vi "main OP300.vi"() -> ()   [LabVIEW 2020]
uses:
  SubVI/OP300ZP_state.ctl
  <vilib>/Sylvain.lib/02 SLIM ZEN WS 500/SubVi/FGV.ctl
  <vilib>/Sylvain.lib/02 SLIM ZEN WS 500/SubVi/VG_progressBar.vi
  SubVI/CheminDeBase.vi
  VG/PN.vi
  VG/IS30%.vi
panel:
  out "IS30% ?":bool
  out "Cluster":T1
  out "VISA OUT":T2
  out "progression":u8(slide) scale=0.0..100.0
  out "PN":string
  out "errout 2":errorcluster={"status"=TRUE, "code"=0, "source"="PCAN_CHANNEL ILLEGAL"} caption="errout"
  out "errout":errorcluster caption="sortie d'erreur"
  out "STOP":bool
  out "TOP":string
  out "DRAW":picture
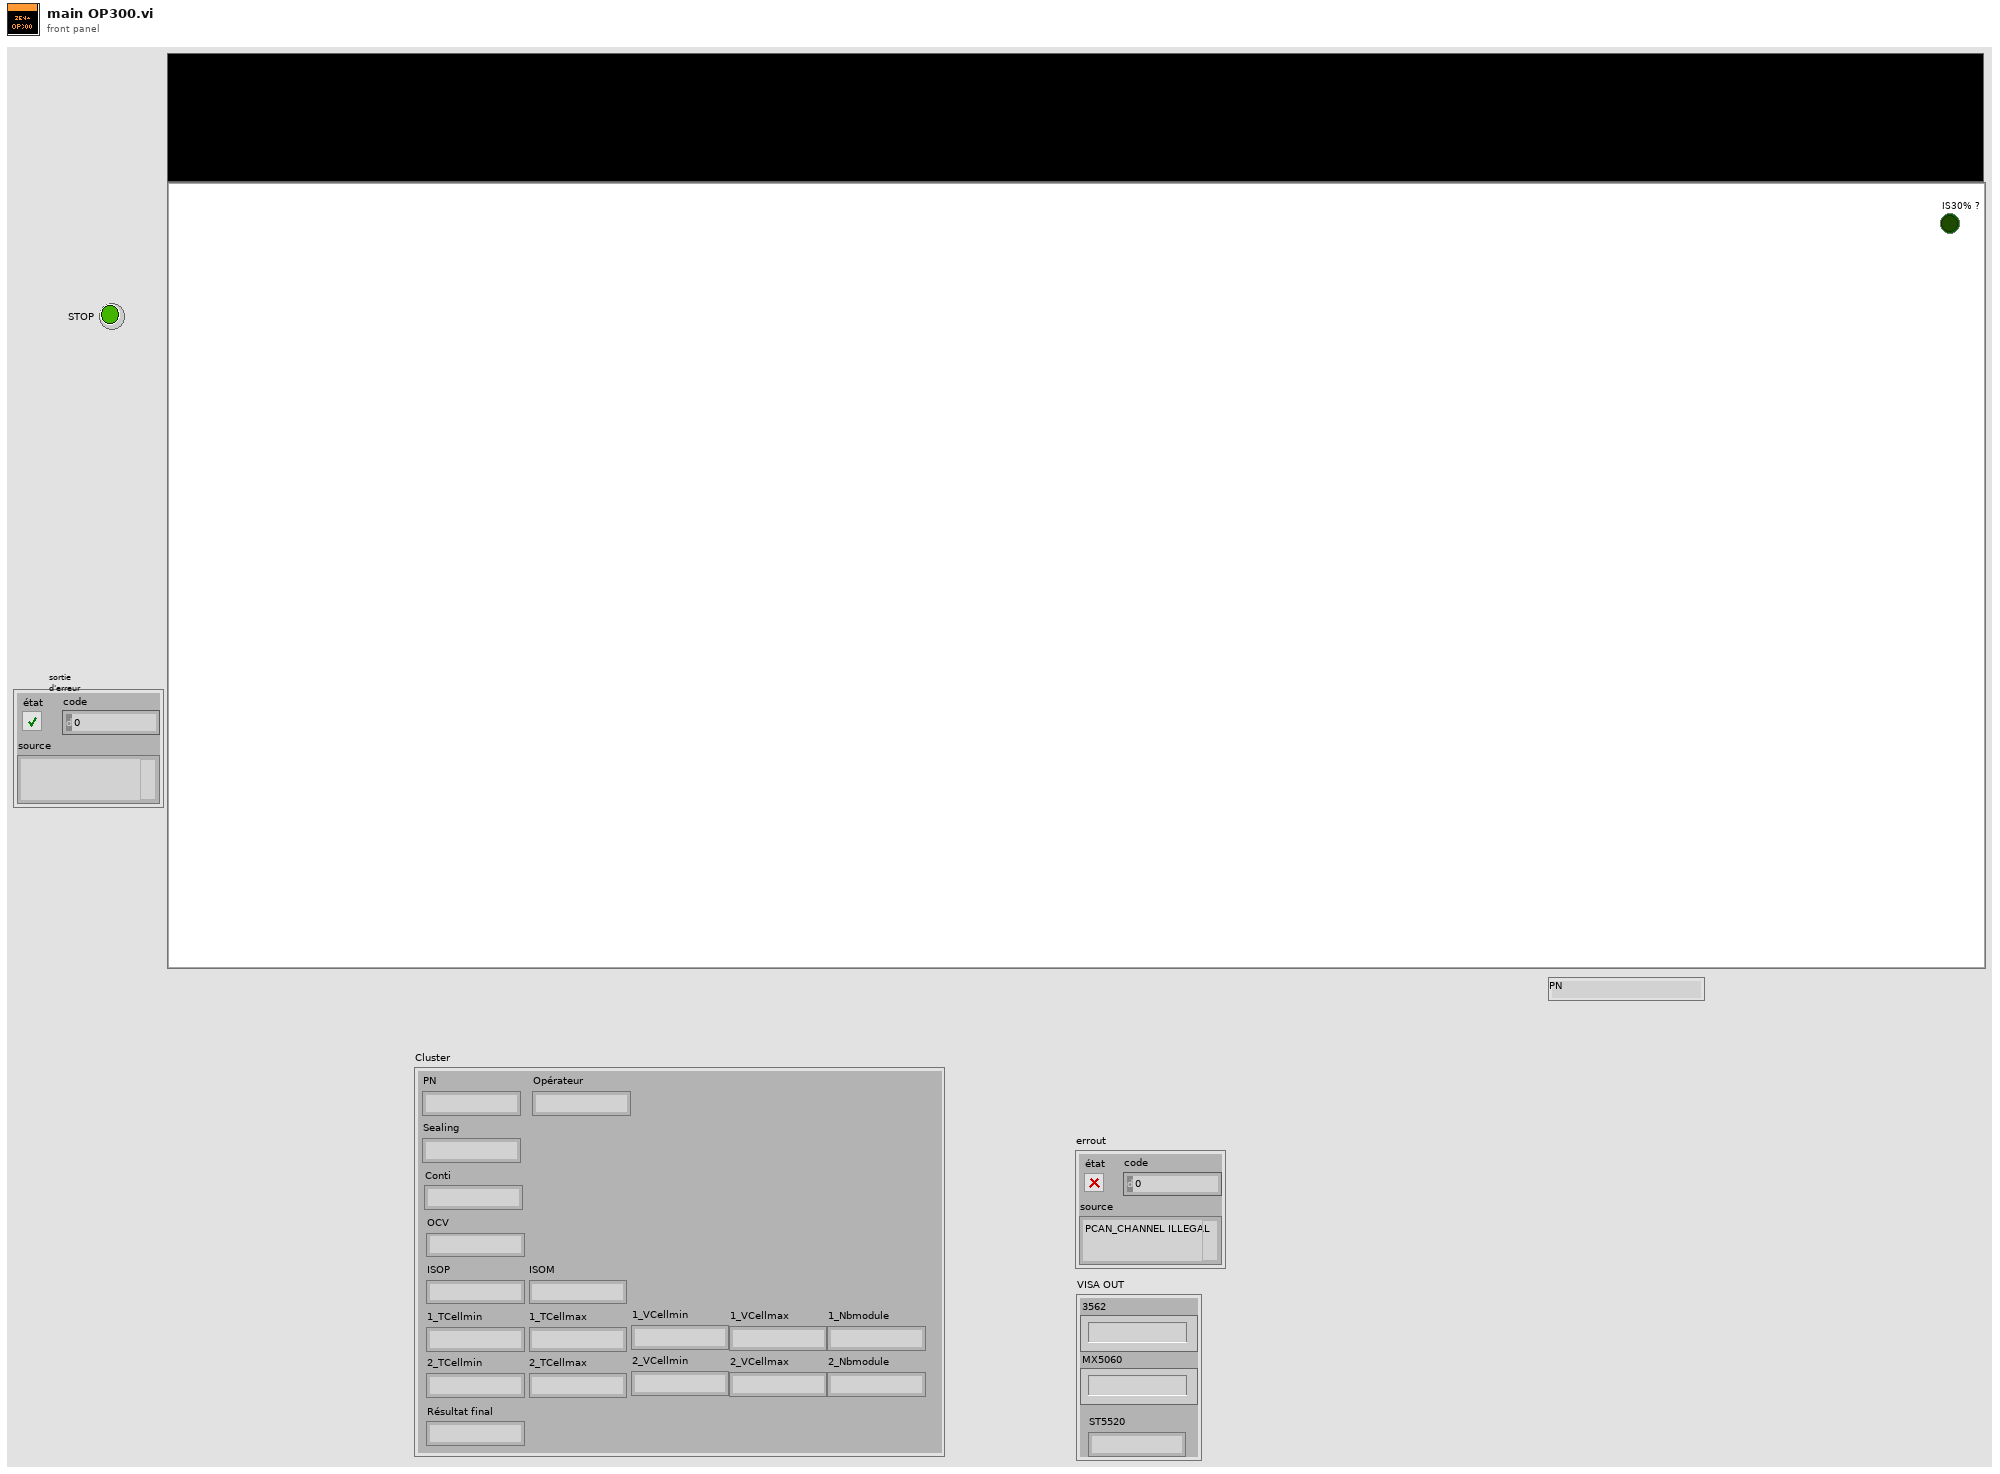
[diagram p1: front panel]
types:
  T1 = cluster{"PN":string, "Opérateur":string, "Sealing":string, "Conti":string, "OCV":string, "ISOP":string, "ISOM":string, "1_TCellmin":string, "1_TCellmax":string, "1_VCellmin":string, "1_VCellmax":string, "1_Nbmodule":string, "2_TCellmin":string, "2_TCellmax":string, "2_VCellmin":string, "2_VCellmax":string, "2_Nbmodule":string, "Résultat final":string}
  T2 = cluster{"3562":string, "MX5060":string, "ST5520":string}
  T3 = cluster{"PN":string, "Sealing":string, "Opérateur":string, "Conti":string, "OCV":string, "ISOP":string, "ISOM":string, "1_TCellmin":string, "1_TCellmax":string, "1_VCellmin":string, "1_VCellmax":string, "1_Nbmodule":string, "2_TCellmin":string, "2_TCellmax":string, "2_VCellmin":string, "2_VCellmax":string, "2_Nbmodule":string, "Résultat final":string}
  T4 = typedef "OP300ZP_state.ctl" = enum16{"Null", "Demarrage", "Init", "Scan", "Montage", "Conti", "OCV", "Iso", "Vpack", "DataDyn", "Dessouter", "DataDyn2", "Demontage", "Crash", "Next", "Sealing", "Comext"}
  T5 = typedef "FGV.ctl" = enum16{"GET", "SET", "RAZ"}
  T6 = cluster{"1_TCellmin":string, "1_TCellmax":string, "1_VCellmin":string, "1_VCellmax":string, "1_Nbmodule":string}
  T7 = cluster{"Chaîne":string, "Chaîne":string, "Chaîne":string, "Chaîne":string, "Chaîne":string, "Chaîne":string, "Chaîne":string, "Chaîne 2":string}
  T8 = typedef "imagedata.ctl" = cluster{"image type":i32, "image depth":i32, "image":u8[], "mask":u8[], "colors":u32[], "Rectangle":cluster{"left":i16, "top":i16, "right":i16, "bottom":i16}}
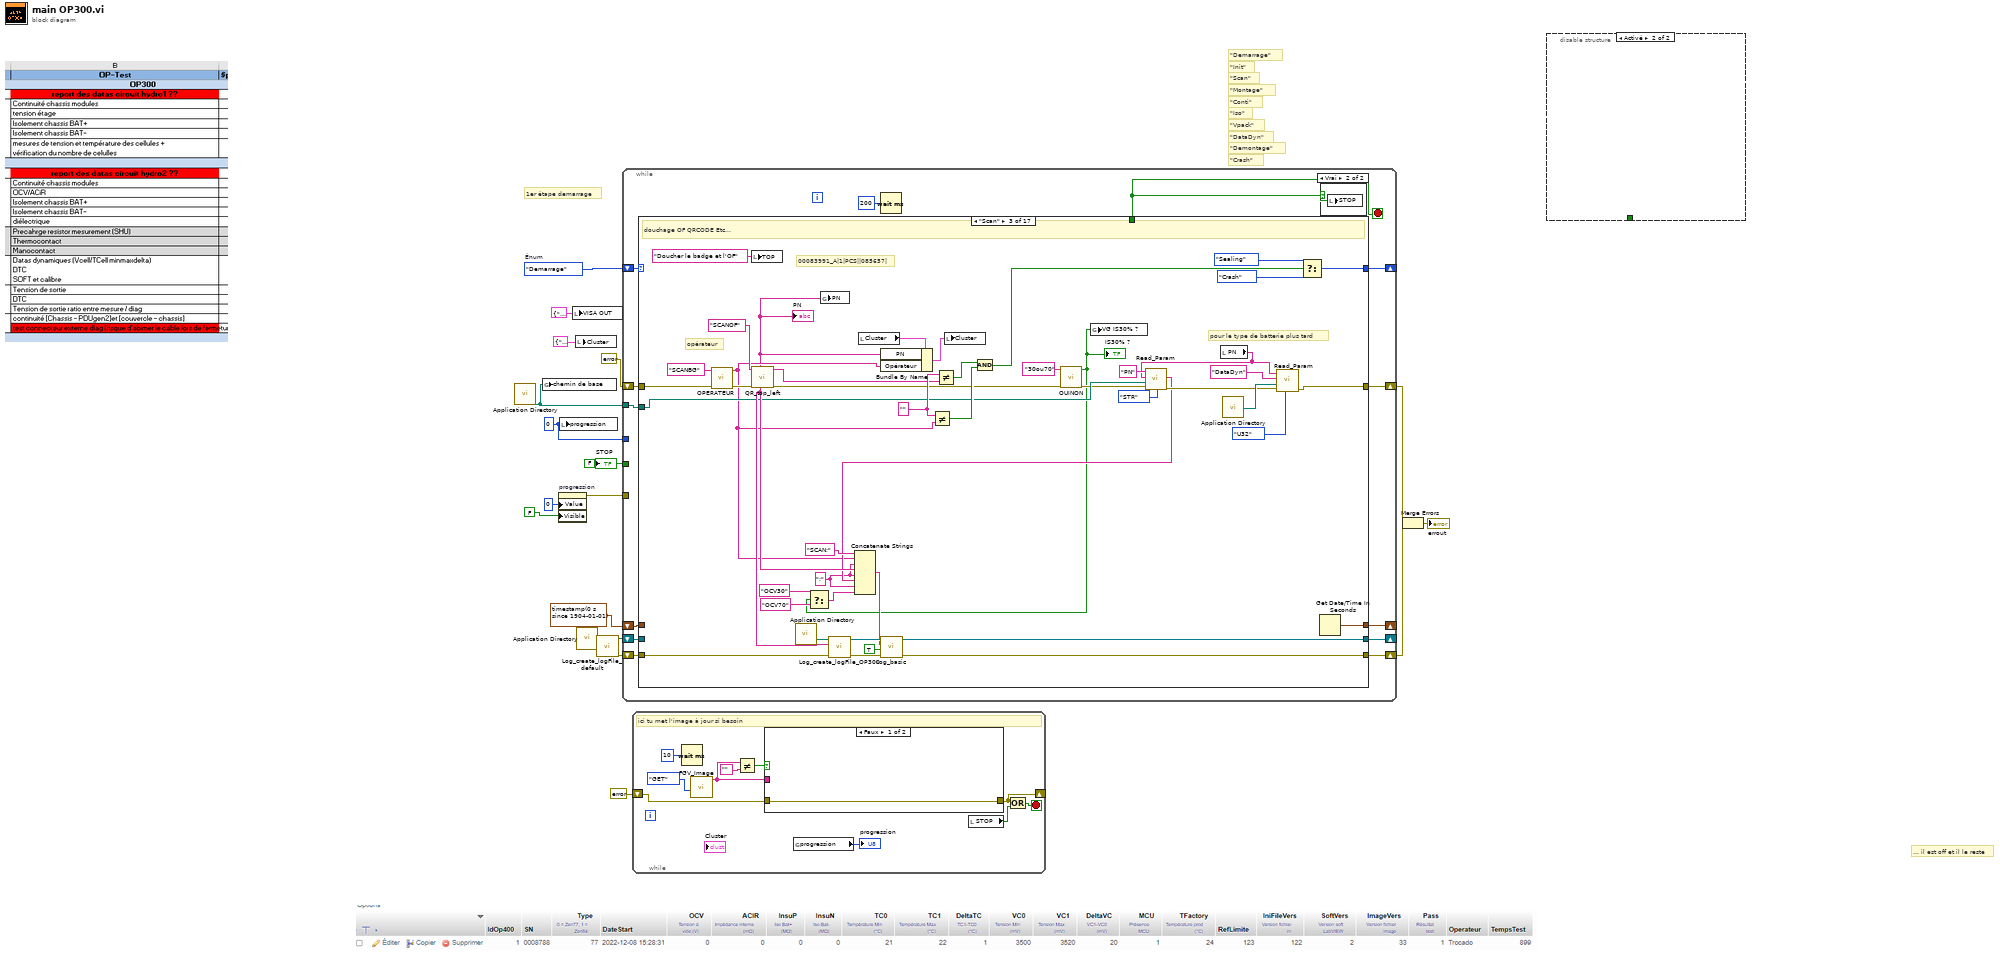
[diagram p0: block diagram]
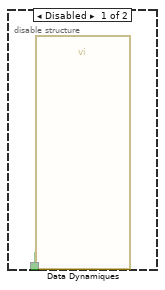
[diagram p2: hidden frame]
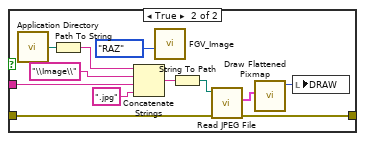
[diagram p3: hidden frame]
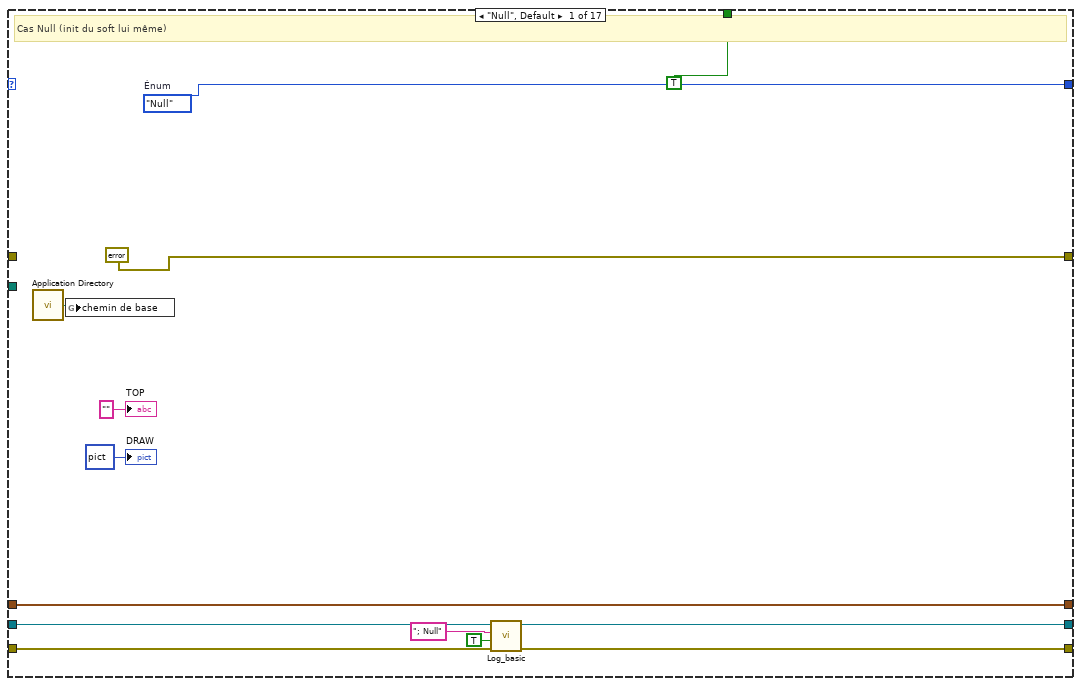
[diagram p5: hidden frame]
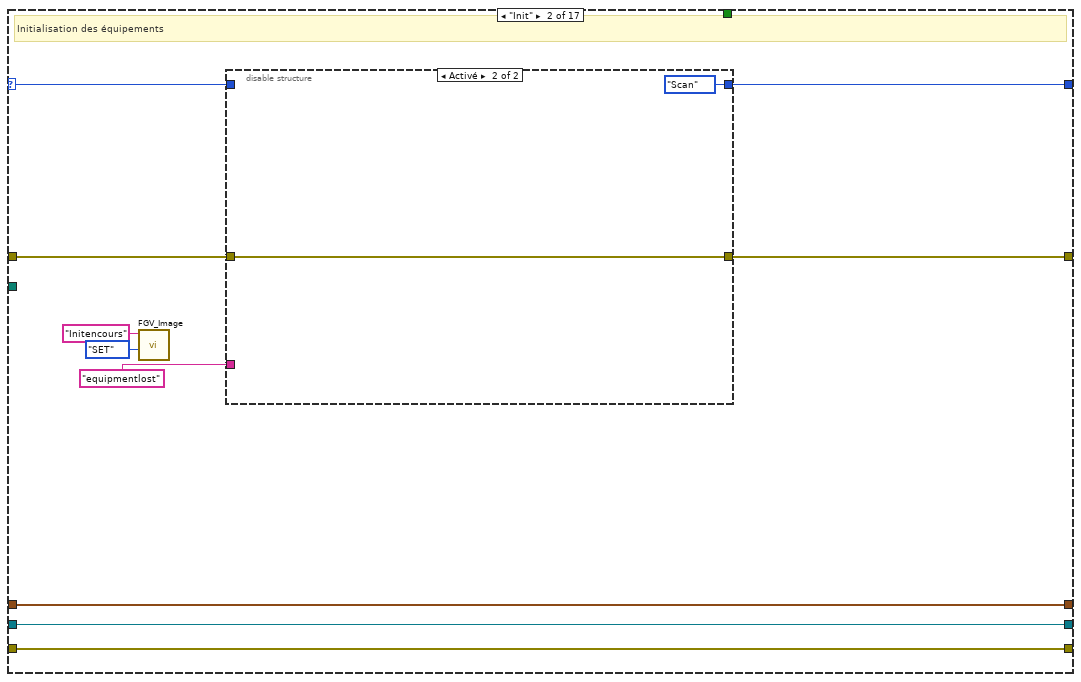
[diagram p6: hidden frame]
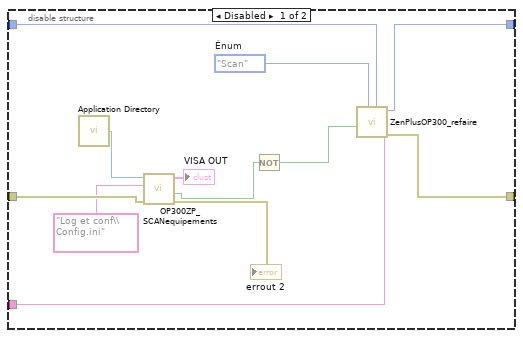
[diagram p7: hidden frame]
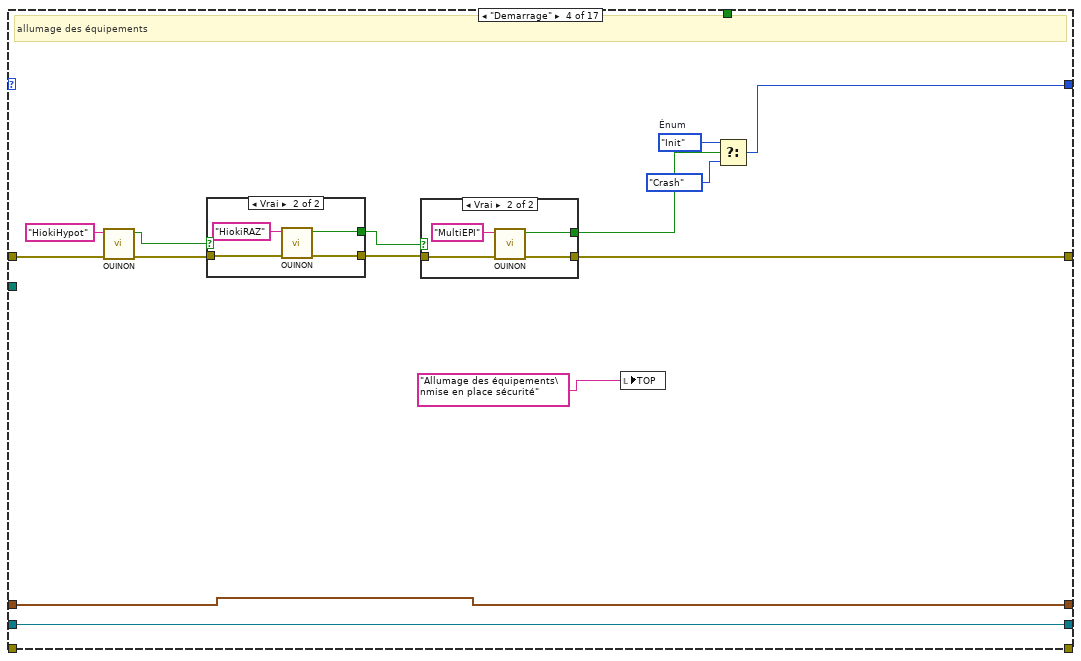
[diagram p8: hidden frame]
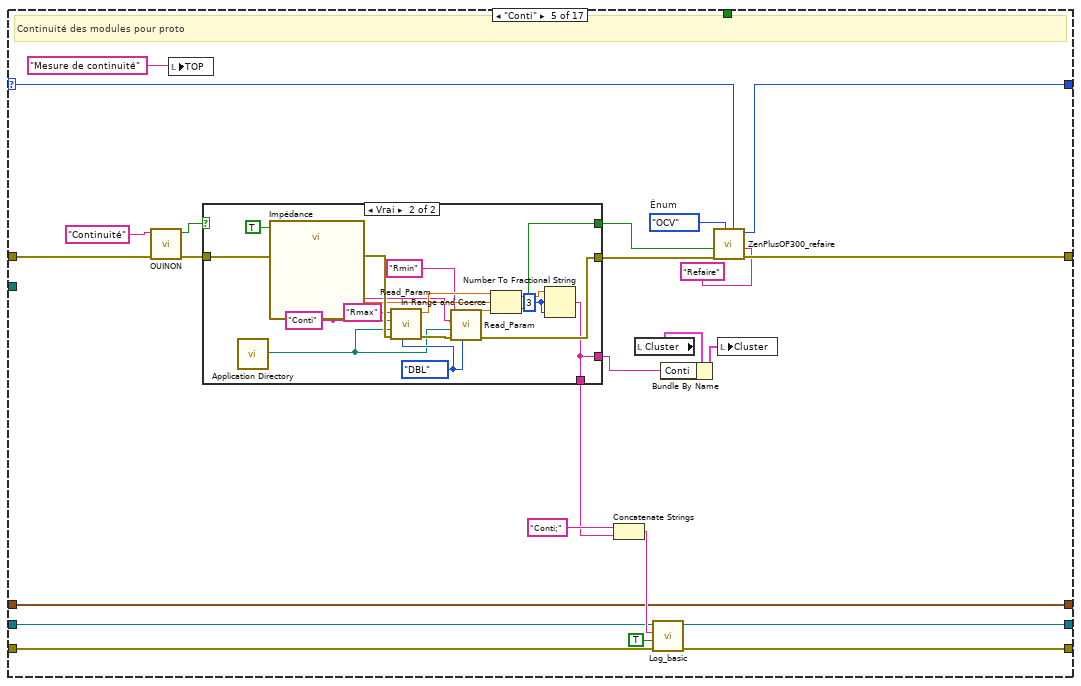
[diagram p11: hidden frame]
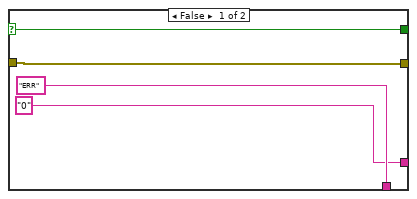
[diagram p12: hidden frame]
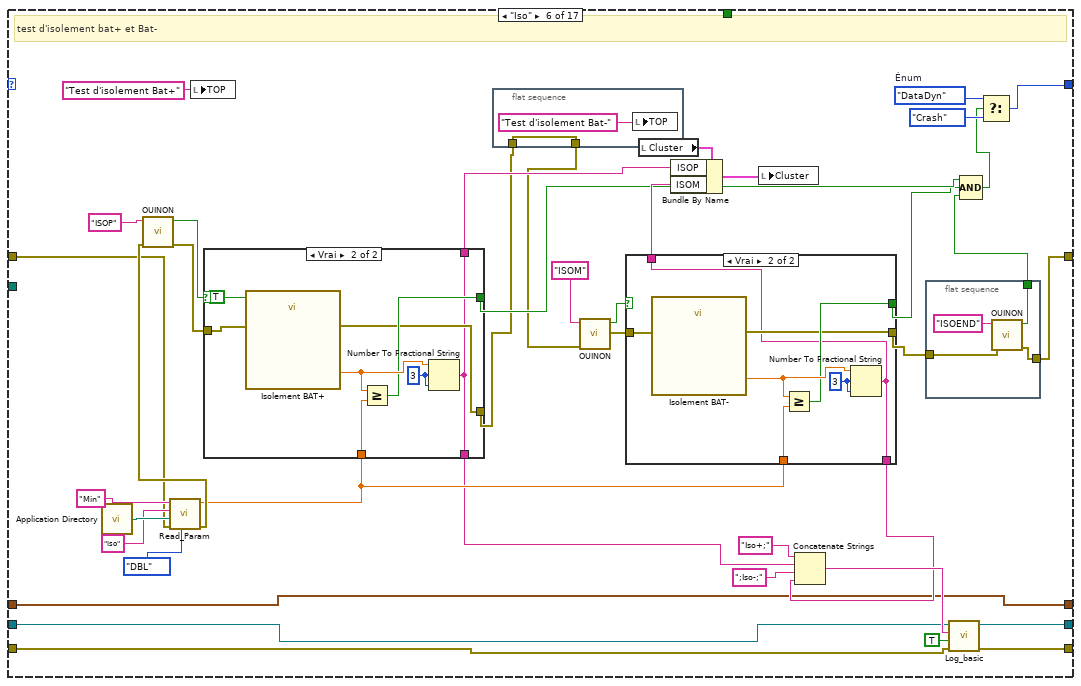
[diagram p13: hidden frame]
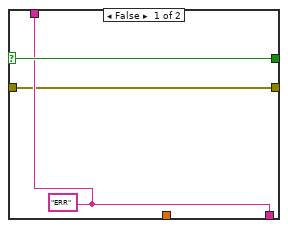
[diagram p14: hidden frame]
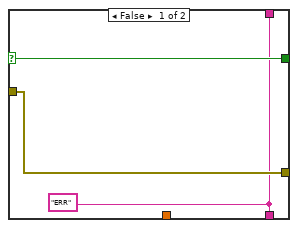
[diagram p15: hidden frame]
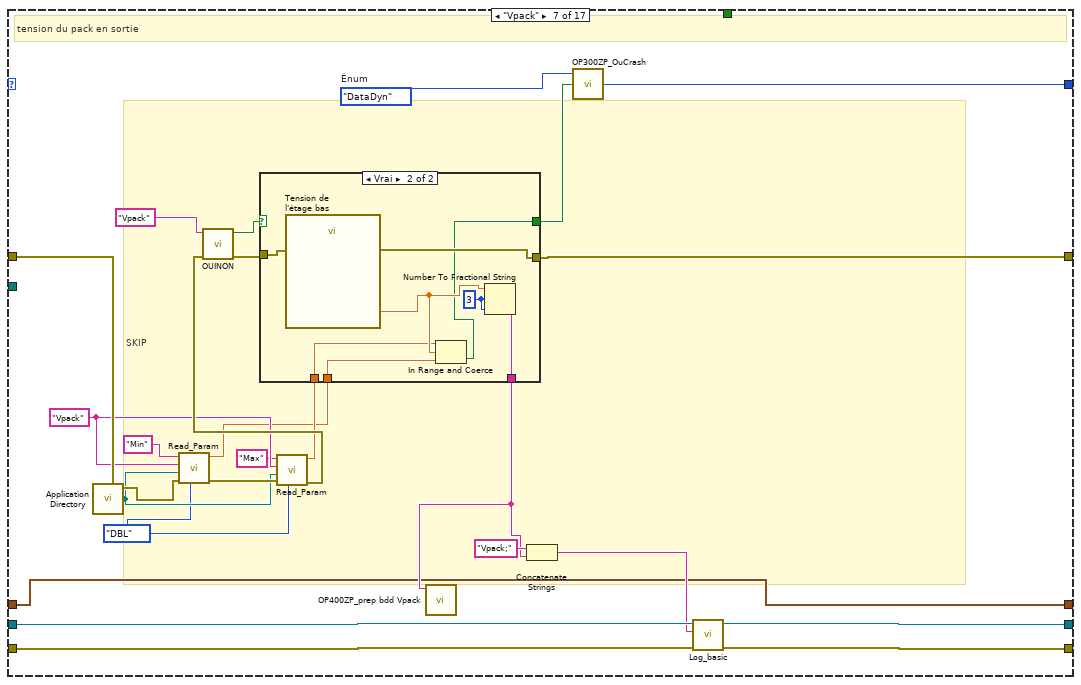
[diagram p16: hidden frame]
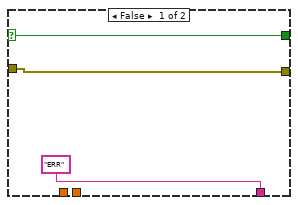
[diagram p17: hidden frame]
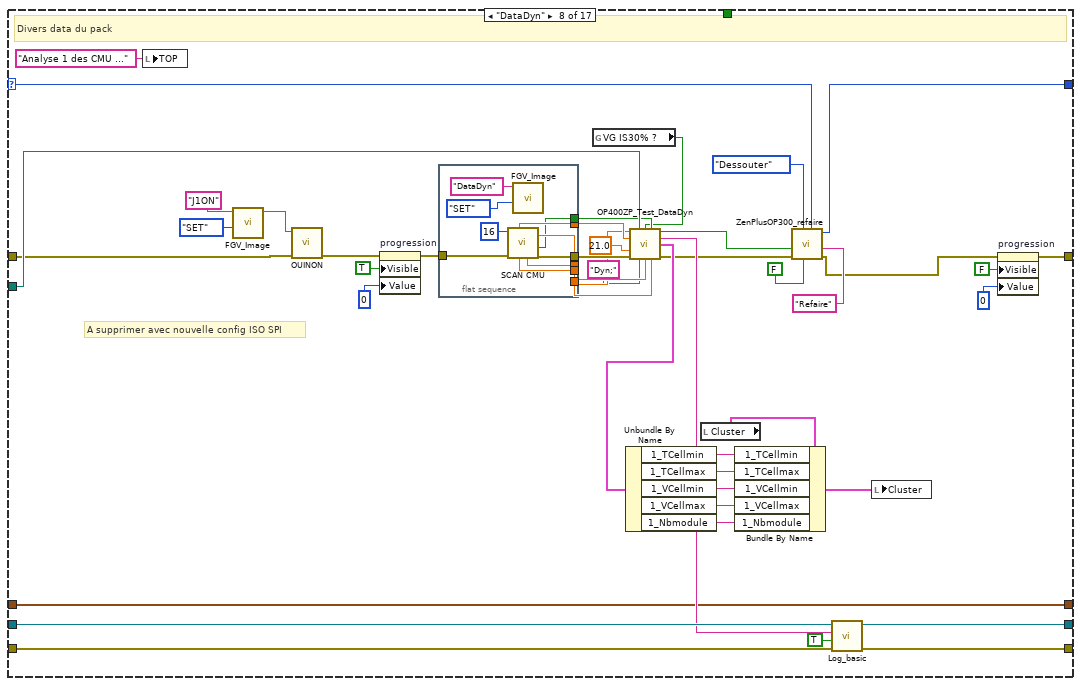
[diagram p18: hidden frame]
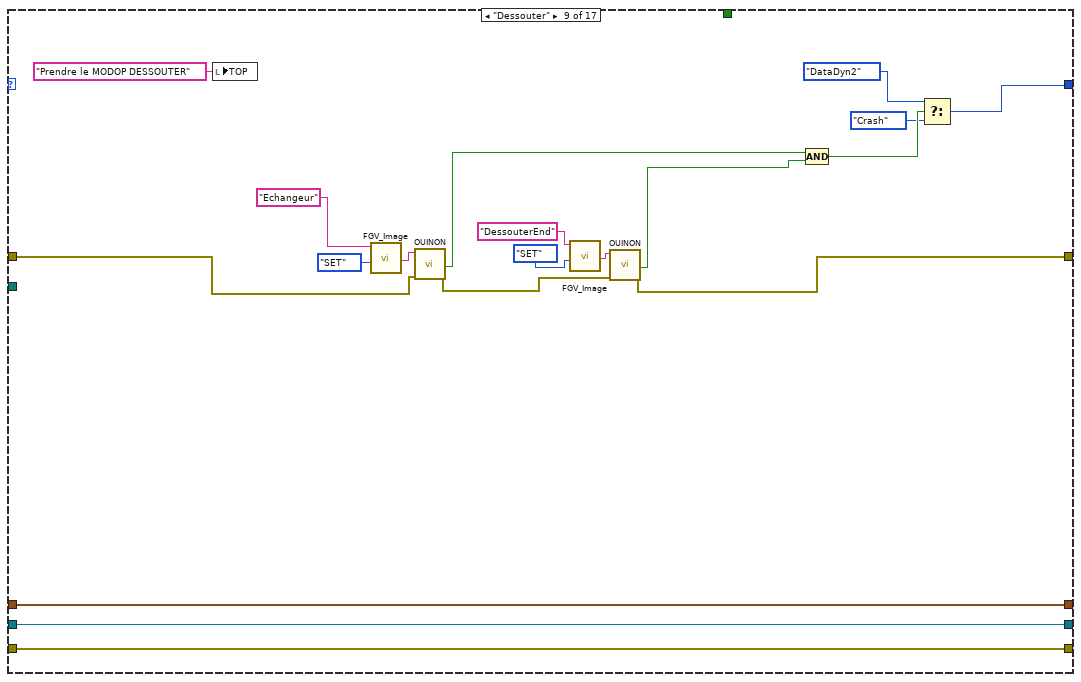
[diagram p19: hidden frame]
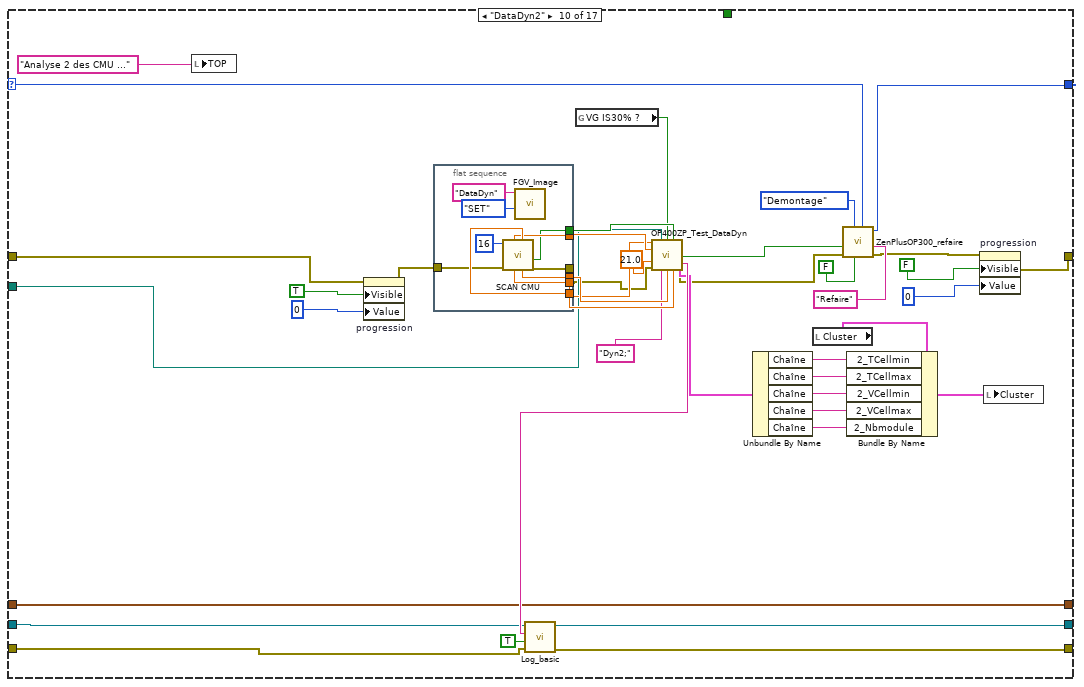
[diagram p20: hidden frame]
diagram:
  w7 = u8 0 ("progression")
  w8 = OP300ZP_state."Demarrage"  # Énum
  w14 = FALSE ("STOP")
  # "1er étape demarrage"
  # "\"Crash\""
  # "\"Demontage\""
  # "\"DataDyn\""
  # "\"Iso\""
  # "\"Montage\""
  # "\"Scan\""
  # "\"Init\""
  # "\"Demarrage\""
  # "\"Conti\""
  # "\"Vpack\""
  # "... il est off et il le reste"
  n1 = call <vilib>:"Application Directory.vi"() -> ("Application Directory"=w13:path)
  n2 = global write "CheminDeBase.vi" "chemin de base"(w13) -> ()
  n3 = property on="progression" class="Gliss (strict)"("Value"=u8 0 ("progression"), "Visible"=FALSE) -> (error out=w5:errorcluster)  [unwired: 2 in, 1 out]
  n4 = local write "progression"(w7) -> ()
  n5 = local write "VISA OUT"(T2 {"3562"="", "MX5060"="", "ST5520"=""} ("VISA OUT")) -> ()
  n6 = local write "Cluster"(T3 {"PN"="0", "Sealing"="0", "Opérateur"="0", "Conti"="0", "OCV"="0", "ISOP"="0", "ISOM"="0", "1_TCellmin"="0", "1_TCellmax"="0", "1_VCellmin"="0", "1_VCellmax"="0", "1_Nbmodule"="0", "2_TCellmin"="0", "2_TCellmax"="0", "2_VCellmin"="0", "2_VCellmax"="0", "2_Nbmodule"="0", "Résultat final"="0"} ("Cluster")) -> ()
  n7 = call <vilib>:"Application Directory.vi"() -> ("Application Directory"=w11:path)
  n8 = call <vilib>:"Log_create_logFile_default.vi"("appdir"=w11) -> ("errout"=w12:errorcluster, "Fichier à flux d'octets en sortie"=w15:refnum<file>)  [unwired: 9 in]
  n9 = while {
    shift-right: [w30] -> w17
    shift-left: errorcluster {"status"=FALSE, "code"=0, "source"=""} ("error out") -> [w19]
    shift-right: [w23] -> _
    shift-left: w8 -> [w24]
    shift-right: [w26] -> w16
    shift-left: w12 -> [w29]
    shift-right: [w27] -> _
    shift-left: w15 -> [w28]
    tunnel: w13 -> [w22]
    tunnel: w14 -> [_]
    shift-right: [w20] -> _
    shift-left: timestamp(0 s since 1904-01-01) ("seconds since 1Jan1904") -> [w21]
    tunnel: w7 -> [_]
    tunnel: w5 -> [_]
    stop <- w25 stop-if-true
    n10 = case shown="\"Scan\"" w24 {
      selector: w24 -> [_ w49 _ _ w148 _ _ w320 _ w386 _ _ _ _ _ w559 w612]
      tunnel: w19 -> [_ w52 w115 w128 w165 w187 w268 w308 w348 w368 w424 w433 w458 w477 w524 w555 w633]
      tunnel: [errorcluster {"status"=FALSE, "code"=0, "source"=""} ("errin") w51 w94 w127 w150 w199 w272 w312 w356 w379 w423 w432 w458 w475 w529 w558 w619] -> w30
      tunnel: w29 -> [w41 w55 w111 _ w159 w213 w278 w333 w347 w382 w421 w435 w461 w500 w538 w564 w622]
      tunnel: w28 -> [w42 w54 _ w129 w158 w212 w277 w334 w345 w384 w422 w436 w462 w501 w537 w563 w624]
      tunnel: [w39 w54 w113 w129 w157 w211 w276 w331 w345 w380 w422 w436 _ _ w536 w562 w620] -> w27
      tunnel: [w40 w55 w114 _ w156 w214 w275 w332 w347 w381 w421 w435 w450 w493 w512 w561 w621] -> w26
      tunnel: [TRUE _ _ _ _ _ _ _ _ _ _ FALSE w463 _ _ _ _] -> w25
      tunnel: [w33 w50 w83 w116 w149 w206 w273 w294 w350 w387 w419 w427 OP300ZP_state."Crash" w502 w528 w560 w617] -> w23
      tunnel: w22 -> [_ _ w88 _ _ _ _ w330 _ w385 _ _ _ _ _ w557 _]
      tunnel: w21 -> [w35 w53 _ w126 w154 w207 w255 w328 w346 w383 w420 w431 _ _ w525 w552 w623]
      tunnel: [w35 w53 w102 w126 w154 w207 w255 w328 w346 w383 w420 w431 _ _ w525 w553 w623] -> w20
      frame "Null", Default {
        w33 = OP300ZP_state."Null"  # Énum
        # "Cas Null (init du soft lui même)"
        n11 = call <vilib>:"Application Directory.vi"() -> ("Application Directory"=w45:path)
        n12 = global write "CheminDeBase.vi" "chemin de base"(w45) -> ()
        n13 = call <vilib>:"Log_basic.vi"("errin"=w41, "date?"=TRUE, "chaîne"="; Null", "in"=w42) -> ("sortie d'erreur"=w40:errorcluster, "refnum en sortie"=w39:refnum<file>)  [unwired: 6 in]
        "DRAW" <- picture data[5B] ("DRAW")
        "TOP" <- "" ("TOP")
      }
      frame "Init" {
        # "Initialisation des équipements"
        n14 = call <vilib>:"FGV_Image.vi"("Énum"=FGV."SET", "IN"="Initencours") -> ()  [unwired: 9 in, 1 out]
        n15 = disable-structure shown="Activé" {
          disable-tunnel: w52 -> [w67 w69]
          disable-tunnel: [w62 w69] -> w51
          disable-tunnel: [w61 OP300ZP_state."Scan" ("Next")] -> w50
          disable-tunnel: w49 -> [w60 _]
          disable-tunnel: "equipmentlost" ("image") -> [w58 _]
          frame Disabled {
            w59 = OP300ZP_state."Scan"  # Énum
            n16 = call <vilib>:"Application Directory.vi"() -> ("Application Directory"=w65:path)
            n17 = call "OP300ZP_SCANequipements.vi"("Errin"=w67, "Chaîne"="Log et conf\\Config.ini", "pathin"=w65) -> ("errout"=→"errout 2":errorcluster, "KO?"=w63:bool, "VISA OUT"=→"VISA OUT":T2)  [unwired: 6 in]
            n18 = Not(x=w63) -> (.not. x?=w64:bool)
            n19 = call "ZenPlusOP300_refaire.vi"("image"=w58, "refaire"=w60, "casOK"=w59, "test ok ?"=w64) -> ("errout"=w62:errorcluster, "Next"=w61:T4)  [unwired: 6 in]
          }
          frame Enabled {
          }
        }
      }
      frame "Scan" {
        w73 = ";" ("chaîne")
        w105 = "" ("x")
        # "pour le type de batterie plus tard"
        # "00083991_A|1|PCS||085657|"
        # "opérateur"
        # "douchage OF QRCODE Etc..."
        n20 = call <vilib>:"OPERATEUR.vi"("errin"=w115, "IN"="SCANBG") -> ("error out"=w101:errorcluster, "Dataout"=w79:string)  [unwired: 8 in]
        n21 = local write "TOP"("Doucher le badge et l'OF" ("TOP")) -> ()
        n22 = call <vilib>:"QR_top_left.vi"("errin"=w101, "image"="SCANOF") -> ("error out"=w77:errorcluster, "Réponse"=w99:string, "SN"=w98:string, "PN"=w70:string)  [unwired: 5 in, 1 out]
        "PN" <- w70
        n23 = call <vilib>:"Application Directory.vi"() -> ("Application Directory"=w112:path)
        n24 = global write "PN.vi" "PN"(w70) -> ()
        n25 = call "Log_create_logFile_OP300.vi"("errin"=w111, "toute l'expression"=w98, "Application Directory"=w112) -> ("sortie d'erreur"=w109:errorcluster, "Fichier à flux d'octets en sortie"=w110:refnum<file>)  [unwired: 7 in]
        n26 = local read "Cluster"() -> (w81:T1)
        n27 = Bundle By Name(cluster=w81, "PN"=w70, "Opérateur"=w79) -> (w80:T1)
        n28 = Not Equal?(x=w105, y=w79) -> (x != y?=w103:bool)
        n29 = Not Equal?(x=w105, y=w99) -> (x != y?=w104:bool)
        n30 = local write "Cluster"(w80) -> ()
        n31 = Compound Arithmetic op=AND ("Opérateur arithmétique")(w104, w103) -> (w86:bool)
        n32 = call <vilib>:"OUINON.vi"("errin"=w77, "image"="30ou70") -> ("error out"=w76:errorcluster, "OUI/NON"=w71:bool)  [unwired: 8 in]
        "IS30% ?" <- w71
        n33 = Select ("Sélectionner")(t="OCV30" ("section"), s=w71, f="OCV70" ("section")) -> (s? t:f=w72:string)
        n34 = global write "IS30%.vi" "VG IS30% ?"(w71) -> ()
        n35 = local read "PN"() -> (w90:string)
        n36 = call <vilib>:"Read_Param.vi"("Énum"=enum16{"STR", "DBL", "U32"}."STR", "errin"=w76, "pathin"=w88, "section"=w90, "key"="PN") -> ("error out"=w93:errorcluster, "str"=w89:string)  [unwired: 2 in, 3 out]
        n37 = Concatenate Strings("SCAN;" ("chaîne"), w79, w73, w98, w73, w89, w73, w72) -> (w107:string)
        n38 = call <vilib>:"Log_basic.vi"("errin"=w109, "date?"=TRUE, "chaîne"=w107, "in"=w110) -> ("sortie d'erreur"=w114:errorcluster, "refnum en sortie"=w113:refnum<file>)  [unwired: 6 in]
        n39 = call <vilib>:"Application Directory.vi"() -> ("Application Directory"=w97:path)
        n40 = call <vilib>:"Read_Param.vi"("Énum"=enum16{"STR", "DBL", "U32"}."U32", "errin"=w93, "pathin"=w97, "section"="DataDyn", "key"=w90) -> ("error out"=w94:errorcluster)  [unwired: 2 in, 4 out]
        n41 = Select ("Sélectionner")(t=OP300ZP_state."Sealing" ("Énum"), s=w86, f=OP300ZP_state."Crash" ("cas faux")) -> (s? t:f=w83:T4)
        n42 = Get Date/Time In Seconds() -> (seconds since 1Jan1904=w102:timestamp)
      }
      frame "Demarrage" {
        w118 = OP300ZP_state."Init"  # Énum
        # "allumage des équipements"
        n43 = call <vilib>:"OUINON.vi"("errin"=w128, "image"="HiokiHypot") -> ("error out"=w124:errorcluster, "OUI/NON"=w121:bool)  [unwired: 8 in]
        n44 = case shown="Vrai" w121 {
          selector: w121 -> [w131 _]
          tunnel: [w131 w135] -> w122
          tunnel: [w130 w134] -> w123
          tunnel: w124 -> [w130 w132]
          frame False {
          }
          frame True {
            n45 = call <vilib>:"OUINON.vi"("errin"=w132, "image"="HiokiRAZ" ("IN")) -> ("error out"=w134:errorcluster, "OUI/NON"=w135:bool)  [unwired: 8 in]
          }
        }
        n46 = case shown="Vrai" w122 {
          selector: w122 -> [w137 _]
          tunnel: [w137 w141] -> w119
          tunnel: [w136 w140] -> w127
          tunnel: w123 -> [w136 w138]
          frame False {
          }
          frame True {
            n47 = call <vilib>:"OUINON.vi"("errin"=w138, "image"="MultiEPI" ("IN")) -> ("error out"=w140:errorcluster, "OUI/NON"=w141:bool)  [unwired: 8 in]
          }
        }
        n48 = local write "TOP"("Allumage des équipements\nmise en place sécurité" ("TOP")) -> ()
        n49 = Select ("Sélectionner")(t=w118, s=w119, f=OP300ZP_state."Crash" ("cas faux")) -> (s? t:f=w116:T4)
      }
      frame "Conti" {
        w147 = OP300ZP_state."OCV"  # Énum
        # "Continuité des modules pour proto"
        n50 = call <vilib>:"OUINON.vi"("errin"=w165, "image"="Continuité" ("IN")) -> ("error out"=w162:errorcluster, "OUI/NON"=w163:bool)  [unwired: 8 in]
        n51 = local write "TOP"("Mesure de continuité" ("TOP")) -> ()
        n52 = case shown="Vrai" w163 {
          selector: w163 -> [w167 _]
          tunnel: w162 -> [w169 w186]
          tunnel: [w169 w182] -> w151
          tunnel: ["ERR" w170] -> w153
          tunnel: [w167 w174] -> w146
          tunnel: ["0" w170] -> w142
          frame False {
          }
          frame True {
            w175 = i16 3 ("largeur (-)")
            w172 = "Conti" ("section")
            w185 = enum16{"STR", "DBL", "U32"}."DBL" ("Énum")
            n53 = call <vilib>:"Application Directory.vi"() -> ("Application Directory"=w177:path)
            n54 = call "Impédance"("Enable"=TRUE, "error in (no error)"=w186) -> ("Conti"=w179:dbl, "error out"=w183:errorcluster)  [unwired: 15 in, 1 out]
            n55 = call <vilib>:"Read_Param.vi"("Énum"=w185, "errin"=w183, "pathin"=w177, "section"=w172, "key"="Rmax") -> ("error out"=w184:errorcluster, "dbl"=w181:dbl)  [unwired: 2 in, 3 out]
            n56 = call <vilib>:"Read_Param.vi"("Énum"=w185, "errin"=w184, "pathin"=w177, "section"=w172, "key"="Rmin") -> ("error out"=w182:errorcluster, "dbl"=w180:dbl)  [unwired: 2 in, 3 out]
            n57 = In Range and Coerce(upper limit=w181, x=w179, lower limit=w180) -> (coerced(x)=w176:dbl, In Range?=w174:bool)
            n58 = Number To Fractional String(number=w176, width (-)=w175, precision (6)=w175) -> (F-format string=w170:string)  [unwired: 1 in]
          }
        }
        n59 = Concatenate Strings("Conti;" ("chaîne"), w153) -> (w161:string)
        n60 = local read "Cluster"() -> (w144:T1)
        n61 = call <vilib>:"Log_basic.vi"("errin"=w159, "date?"=TRUE, "chaîne"=w161, "in"=w158) -> ("sortie d'erreur"=w156:errorcluster, "refnum en sortie"=w157:refnum<file>)  [unwired: 6 in]
        n62 = Bundle By Name(cluster=w144, "Conti"=w142) -> (w143:T1)
        n63 = call "ZenPlusOP300_refaire.vi"("image"="Refaire", "refaire"=w148, "casOK"=w147, "errin"=w151, "test ok ?"=w146) -> ("errout"=w150:errorcluster, "Next"=w149:T4)  [unwired: 5 in]
        n64 = local write "Cluster"(w143) -> ()
      }
      frame "Iso" {
        w205 = OP300ZP_state."DataDyn"  # Énum
        # "test d'isolement bat+ et Bat-"
        n65 = call <vilib>:"Application Directory.vi"() -> ("Application Directory"=w222:path)
        n66 = call <vilib>:"Read_Param.vi"("Énum"=enum16{"STR", "DBL", "U32"}."DBL", "errin"=w187, "pathin"=w222, "section"="Iso", "key"="Min") -> ("error out"=w219:errorcluster, "dbl"=w216:dbl)  [unwired: 2 in, 3 out]
        n67 = call <vilib>:"OUINON.vi"("errin"=w219, "image"="ISOP" ("IN")) -> ("error out"=w192:errorcluster, "OUI/NON"=w193:bool)  [unwired: 8 in]
        n68 = local write "TOP"("Test d'isolement Bat+" ("TOP")) -> ()
        n69 = case shown="Vrai" w193 {
          selector: w193 -> [w244 _]
          tunnel: w192 -> [w245 w253]
          tunnel: [w245 w248] -> w190
          tunnel: [w243 w247] -> w209
          tunnel: [w244 w249] -> w197
          tunnel: w216 -> [_ w251]
          tunnel: [w243 w247] -> w201
          frame False {
            w243 = "ERR"
          }
          frame True {
            w252 = i16 3 ("largeur (-)")
            n70 = call "Isolement BAT+"("Enable"=TRUE, "error in (no error)"=w253) -> ("ISOP"=w250:dbl, "error out"=w248:errorcluster)  [unwired: 15 in, 1 out]
            n71 = Greater Or Equal?(x=w250, y=w251) -> (x >= y?=w249:bool)
            n72 = Number To Fractional String(number=w250, width (-)=w252, precision (6)=w252) -> (F-format string=w247:string)  [unwired: 1 in]
          }
        }
        n73 = flat-sequence {
          tunnel: w190 -> [w227]
          tunnel: [w227] -> w189
          frame #0 {
            n74 = local write "TOP"("Test d'isolement Bat-" ("TOP")) -> ()
          }
        }
        n75 = call <vilib>:"OUINON.vi"("errin"=w189, "image"="ISOM" ("IN")) -> ("error out"=w191:errorcluster, "OUI/NON"=w217:bool)  [unwired: 8 in]
        n76 = case shown="Vrai" w217 {
          selector: w217 -> [w235 _]
          tunnel: [w233 w238] -> w198
          tunnel: [w234 w237] -> w208
          tunnel: [w235 w239] -> w196
          tunnel: w216 -> [_ w241]
          tunnel: [w234 w237] -> w200
          tunnel: w191 -> [w233 w236]
          frame False {
            w234 = "ERR"
          }
          frame True {
            w242 = i16 3 ("largeur (-)")
            n77 = call "Isolement BAT-"("error in (no error)"=w236) -> ("ISOM"=w240:dbl, "error out"=w238:errorcluster)  [unwired: 16 in, 1 out]
            n78 = Greater Or Equal?(x=w240, y=w241) -> (x >= y?=w239:bool)
            n79 = Number To Fractional String(number=w240, width (-)=w242, precision (6)=w242) -> (F-format string=w237:string)  [unwired: 1 in]
          }
        }
        n80 = local read "Cluster"() -> (w203:T1)
        n81 = Bundle By Name(cluster=w203, "ISOP"=w201, "ISOM"=w200) -> (w202:T1)
        n82 = local write "Cluster"(w202) -> ()
        n83 = Concatenate Strings("Iso+;" ("chaîne"), w209, ";Iso-;" ("chaîne"), w208) -> (w225:string)
        n84 = flat-sequence {
          tunnel: [w230] -> w199
          tunnel: w198 -> [w231]
          tunnel: [w229] -> w195
          frame #0 {
            n85 = call <vilib>:"OUINON.vi"("errin"=w231, "image"="ISOEND") -> ("error out"=w230:errorcluster, "OUI/NON"=w229:bool)  [unwired: 8 in]
          }
        }
        n86 = call <vilib>:"Log_basic.vi"("errin"=w213, "date?"=TRUE, "chaîne"=w225, "in"=w212) -> ("sortie d'erreur"=w214:errorcluster, "refnum en sortie"=w211:refnum<file>)  [unwired: 6 in]
        n87 = Compound Arithmetic op=AND ("Opérateur arithmétique")(w197, w196, w195) -> (w194:bool)
        n88 = Select ("Sélectionner")(t=w205, s=w194, f=OP300ZP_state."Crash" ("cas faux")) -> (s? t:f=w206:T4)
      }
      frame "Vpack" {
        w254 = OP300ZP_state."DataDyn"  # Énum
        w263 = enum16{"STR", "DBL", "U32"}."DBL" ("Énum")
        w266 = "Vpack" ("section")
        # "SKIP"
        # "tension du pack en sortie"
        n89 = call <vilib>:"Application Directory.vi"() -> ("Application Directory"=w264:path)
        n90 = call <vilib>:"Read_Param.vi"("Énum"=w263, "errin"=w268, "pathin"=w264, "section"=w266, "key"="Min") -> ("error out"=w269:errorcluster, "dbl"=w261:dbl)  [unwired: 2 in, 3 out]
        n91 = call <vilib>:"Read_Param.vi"("Énum"=w263, "errin"=w269, "pathin"=w264, "section"=w266, "key"="Max") -> ("error out"=w267:errorcluster, "dbl"=w262:dbl)  [unwired: 2 in, 3 out]
        n92 = call <vilib>:"OUINON.vi"("errin"=w267, "image"="Vpack" ("IN")) -> ("error out"=w271:errorcluster, "OUI/NON"=w258:bool)  [unwired: 8 in]
        n93 = case shown="Vrai" w258 {
          selector: w258 -> [w279 _]
          tunnel: w271 -> [w281 w289]
          tunnel: [w281 w286] -> w272
          tunnel: ["ERR" w287] -> w256
          tunnel: [w279 w284] -> w257
          tunnel: w262 -> [_ w282]
          tunnel: w261 -> [_ w283]
          frame False {
          }
          frame True {
            w288 = i16 3 ("largeur (-)")
            n94 = call "Tension de l'étage bas"("error in (no error)"=w289) -> ("Vpack"=w285:dbl, "error out"=w286:errorcluster)  [unwired: 16 in, 1 out]
            n95 = In Range and Coerce(upper limit=w282, x=w285, lower limit=w283) -> (In Range?=w284:bool)  [unwired: 1 out]
            n96 = Number To Fractional String(number=w285, width (-)=w288, precision (6)=w288) -> (F-format string=w287:string)  [unwired: 1 in]
          }
        }
        n97 = call "OP400ZP_prep bdd Vpack.vi"("OCV"=w256) -> ()  [unwired: 10 in, 1 out]
        n98 = Concatenate Strings("Vpack;" ("chaîne"), w256) -> (w259:string)
        n99 = call "OP300ZP_OuCrash.vi"("Booléen"=w257, "in"=w254) -> ("OUT"=w273:T4)  [unwired: 1 in]
        n100 = call <vilib>:"Log_basic.vi"("errin"=w278, "chaîne"=w259, "in"=w277) -> ("sortie d'erreur"=w275:errorcluster, "refnum en sortie"=w276:refnum<file>)  [unwired: 7 in]
      }
      frame "DataDyn" {
        # "A supprimer avec nouvelle config ISO SPI"
        # "Divers data du pack"
        n101 = local write "TOP"("Analyse 1 des CMU ..." ("TOP")) -> ()
        n102 = call <vilib>:"FGV_Image.vi"("Énum"=FGV."SET", "IN"="J1ON") -> ("OUT"=w309:string)  [unwired: 9 in]
        n103 = call <vilib>:"OUINON.vi"("errin"=w308, "image"=w309) -> ("error out"=w307:errorcluster)  [unwired: 8 in, 1 out]
        n104 = property on="progression" class="Gliss (strict)"(error in=w307, "Visible"=TRUE, "Value"=u8 0 ("progression")) -> (error out=w316:errorcluster)  [unwired: 1 in, 1 out]
        n105 = flat-sequence {
          tunnel: [w344] -> w327
          tunnel: [w343] -> w326
          tunnel: [w342] -> w325
          tunnel: [w341] -> w324
          tunnel: [w340] -> w323
          tunnel: [w339] -> w322
          tunnel: w316 -> [w338]
          frame #0 {
            n106 = call "SCAN CMU.vi"("errin"=w338, "Nb modules"=i16 16) -> ("errout"=w344:errorcluster, "# température + #tension OK?"=w339:bool, "Vmin"=w343:dbl, "Vmax"=w342:dbl, "Tmin"=w340:dbl, "Tmax"=w341:dbl)  [unwired: 4 out]
            n107 = call <vilib>:"FGV_Image.vi"("Énum"=FGV."SET", "IN"="DataDyn") -> ()  [unwired: 9 in, 1 out]
          }
        }
        n108 = global read "IS30%.vi" "VG IS30% ?"() -> (w290:bool)
        n109 = call "OP400ZP_Test_DataDyn.vi"("Tcell Min (°C)"=w323, "appdir"=w330, "is30%?"=w290, "MCU"=w322, "Tcell Max (°C)"=w324, "Température usine (°C)"=21.0, "errin"=w327, "testname"="Dyn;", "Vcell Min (V)"=w326, "Vcell Max (V)"=w325) -> ("pass"=w291:bool, "datalog"=w329:string, "Cluster"=w300:T6, "errout"=w292:errorcluster)  [unwired: 1 in, 1 out]
        n110 = Unbundle By Name(w300) -> ("1_TCellmin"=w299:string, "1_TCellmax"=w298:string, "1_VCellmin"=w297:string, "1_VCellmax"=w296:string, "1_Nbmodule"=w295:string)
        n111 = local read "Cluster"() -> (w302:T1)
        n112 = Bundle By Name(cluster=w302, "1_TCellmin"=w299, "1_TCellmax"=w298, "1_VCellmin"=w297, "1_VCellmax"=w296, "1_Nbmodule"=w295) -> (w301:T1)
        n113 = call "ZenPlusOP300_refaire.vi"("image"="Refaire", "refaire"=w320, "Pédale"=FALSE, "casOK"=OP300ZP_state."Dessouter" ("Énum"), "errin"=w292, "test ok ?"=w291) -> ("errout"=w293:errorcluster, "Next"=w294:T4)  [unwired: 4 in]
        n114 = call <vilib>:"Log_basic.vi"("errin"=w333, "date?"=TRUE, "chaîne"=w329, "in"=w334) -> ("sortie d'erreur"=w332:errorcluster, "refnum en sortie"=w331:refnum<file>)  [unwired: 6 in]
        n115 = local write "Cluster"(w301) -> ()
        n116 = property on="progression" class="Gliss (strict)"(error in=w293, "Visible"=FALSE, "Value"=u8 0 ("progression")) -> (error out=w312:errorcluster)  [unwired: 1 in, 1 out]
      }
      frame "Dessouter" {
        n117 = local write "TOP"("Prendre le MODOP DESSOUTER" ("TOP")) -> ()
        n118 = call <vilib>:"FGV_Image.vi"("Énum"=FGV."SET", "IN"="Echangeur") -> ("OUT"=w361:string)  [unwired: 9 in]
        n119 = call <vilib>:"OUINON.vi"("errin"=w348, "image"=w361) -> ("error out"=w357:errorcluster, "OUI/NON"=w354:bool)  [unwired: 8 in]
        n120 = call <vilib>:"FGV_Image.vi"("Énum"=FGV."SET", "IN"="DessouterEnd") -> ("OUT"=w360:string)  [unwired: 9 in]
        n121 = call <vilib>:"OUINON.vi"("errin"=w357, "image"=w360) -> ("error out"=w356:errorcluster, "OUI/NON"=w355:bool)  [unwired: 8 in]
        n122 = Compound Arithmetic op=AND(w354, w355) -> (w353:bool)
        n123 = Select(t=OP300ZP_state."DataDyn2" ("Next"), s=w353, f=OP300ZP_state."Crash" ("cas faux")) -> (s? t:f=w350:T4)
      }
      frame "DataDyn2" {
        n124 = local write "TOP"("Analyse 2 des CMU ..." ("TOP")) -> ()
        n125 = property on="progression" class="Gliss (strict)"(error in=w368, "Visible"=TRUE, "Value"=u8 0 ("progression")) -> (error out=w393:errorcluster)  [unwired: 1 in, 1 out]
        n126 = flat-sequence {
          tunnel: [w414] -> w366
          tunnel: [w413] -> w402
          tunnel: [w412] -> w401
          tunnel: [w411] -> w400
          tunnel: [w410] -> w399
          tunnel: [w409] -> w398
          tunnel: w393 -> [w408]
          frame #0 {
            n127 = call "SCAN CMU.vi"("errin"=w408, "Nb modules"=i16 16) -> ("errout"=w414:errorcluster, "# température + #tension OK?"=w409:bool, "Vmin"=w413:dbl, "Vmax"=w412:dbl, "Tmin"=w410:dbl, "Tmax"=w411:dbl)  [unwired: 4 out]
            n128 = call <vilib>:"FGV_Image.vi"("Énum"=FGV."SET", "IN"="DataDyn") -> ()  [unwired: 9 in, 1 out]
          }
        }
        n129 = global read "IS30%.vi" "VG IS30% ?"() -> (w364:bool)
        n130 = call "OP400ZP_Test_DataDyn.vi"("Tcell Min (°C)"=w399, "appdir"=w385, "is30%?"=w364, "MCU"=w398, "Tcell Max (°C)"=w400, "Température usine (°C)"=21.0, "errin"=w366, "testname"="Dyn2;", "Vcell Min (V)"=w402, "Vcell Max (V)"=w401) -> ("pass"=w365:bool, "datalog"=w404:string, "StrData"=w370:T7, "errout"=w367:errorcluster)  [unwired: 1 in, 1 out]
        n131 = call <vilib>:"Log_basic.vi"("errin"=w382, "date?"=TRUE, "chaîne"=w404, "in"=w384) -> ("sortie d'erreur"=w381:errorcluster, "refnum en sortie"=w380:refnum<file>)  [unwired: 6 in]
        n132 = Unbundle By Name(w370) -> ("Chaîne"=w375:string, "Chaîne"=w374:string, "Chaîne"=w373:string, "Chaîne"=w372:string, "Chaîne"=w371:string)
        n133 = local read "Cluster"() -> (w377:T1)
        n134 = call "ZenPlusOP300_refaire.vi"("image"="Refaire", "refaire"=w386, "Pédale"=FALSE, "casOK"=OP300ZP_state."Demontage" ("Énum"), "errin"=w367, "test ok ?"=w365) -> ("errout"=w389:errorcluster, "Next"=w387:T4)  [unwired: 4 in]
        n135 = Bundle By Name(cluster=w377, "2_TCellmin"=w375, "2_TCellmax"=w374, "2_VCellmin"=w373, "2_VCellmax"=w372, "2_Nbmodule"=w371) -> (w376:T1)
        n136 = property on="progression" class="Gliss (strict)"(error in=w389, "Visible"=FALSE, "Value"=u8 0 ("progression")) -> (error out=w379:errorcluster)  [unwired: 1 in, 1 out]
        n137 = local write "Cluster"(w376) -> ()
      }
      frame "Montage" {
        w417 = OP300ZP_state."Conti"  # Énum
        # "montage du produit sur le banc"
        n138 = local write "TOP"("Montage du pack" ("TOP")) -> ()
        n139 = call <vilib>:"OUINON.vi"("errin"=w424, "image"="Montage" ("IN")) -> ("error out"=w423:errorcluster, "OUI/NON"=w418:bool)  [unwired: 8 in]
        n140 = Select ("Sélectionner")(t=w417, s=w418, f=OP300ZP_state."Crash" ("cas faux")) -> (s? t:f=w419:T4)
      }
      frame "Demontage" {
        w429 = OP300ZP_state."Next"  # Énum
        n141 = call <vilib>:"OUINON.vi"("errin"=w433, "image"="Demontage" ("IN")) -> ("error out"=w432:errorcluster, "OUI/NON"=w430:bool)  [unwired: 8 in]
        n142 = Select ("Sélectionner")(t=w429, s=w430, f=OP300ZP_state."Crash" ("cas faux")) -> (s? t:f=w427:T4)
        n143 = local write "TOP"("Demontage du pack" ("TOP")) -> ()
      }
      frame "Crash" {
        # "\\\\forseepower.com\\fr\\040 Production\\FR7 - Poitiers\\06 Production\\05. Electronique\\Documents Control lib\\Archives\\ZEN PLUS"
        n144 = Close File(refnum=w462, error in=w461) -> (path=w448:path, error out=w453:errorcluster)
        n145 = call <vilib>:"waitXms.vi"("attente (ms)"=u32 300, "errin"=w453) -> ("errout"=w449:errorcluster)  [unwired: 13 in]
        n146 = local read "Cluster"() -> (w442:T1)
        n147 = Read from Text File(file (use dialog)=w448, error in=w449) -> (text=w447:string, error out=w445:errorcluster)  [unwired: 2 in, 2 out]
        n148 = call "OP300ZP_SN_Reader.vi"("Fichier txt"=w447) -> ("SN"=w440:string)  [unwired: 10 in]
        n149 = Unbundle By Name(w442) -> ("PN"=w439:string)
        n150 = call <vilib>:"FGV_Image.vi"("Énum"=FGV."SET", "IN"="TeamLeader") -> ()  [unwired: 9 in, 1 out]
        n151 = Concatenate Strings(w439, "-SN" ("chaîne"), w440) -> (w441:string)
        n152 = call "OP300ZP_NouveauDossier.vi"("entrée d'erreur (pas d'erreur)"=w445, "Nom du repertoire (PN SN)"=w441, "Network before adding a new folder"=path "\\\\forseepower.com\\fr/040 Production/FR7 - Poitiers/06 Production/05. Electronique/Documents Control lib/Archives/ZEN PLUS" ("chemin de la cible (utiliser une boîte de dialogue)")) -> ("sortie d'erreur"=w446:errorcluster, "Network after adding a new folder"=w443:path)  [unwired: 7 in]
        n153 = Copy ("Copier")(8:w446, 10:w443, 11:w448) -> (0:w452:errorcluster)  [unwired: 2 in, 2 out]
        n154 = call "PvgeneratorOP300.vi"("errin"=w452, "network"=w443, "path in"=w448) -> ("sortie d'erreur"=w456:errorcluster, "network out"=w455:path)  [unwired: 5 in, 2 out]
        n155 = call <vilib>:"POP_GOOGLE.vi"("error in"=w456, "chemin"=w455) -> ("error out"=w451:errorcluster)  [unwired: 8 in, 1 out]
        n156 = flat-sequence {
          tunnel: [TRUE] -> w463
          tunnel: w450 -> [_]
          frame #0 {
          }
        }
        n157 = disable-structure shown="Désactivé" {
          disable-tunnel: w451 -> [w467 _]
          disable-tunnel: [w464 _] -> w450
          frame Disabled {
            n158 = Select ("Sélectionner")(t="1", s=FALSE ("sélecteur"), f="0" ("cas faux")) -> (s? t:f=w468:string)
            n159 = local read "Cluster"() -> (w471:T1)
            n160 = Bundle By Name(cluster=w471, "Résultat final"=w468) -> (w466:T1)
            n161 = call "BDD_2.vi"("errin"=w467, "Cluster"=w466) -> ("error out"=w464:errorcluster)  [unwired: 8 in, 1 out]
          }
          frame Enabled {
          }
        }
      }
      frame "Next" {
        w498 = OP300ZP_state."Null"  # Énum
        w499 = OP300ZP_state."Scan"  # Énum
        # "\\\\forseepower.com\\fr\\040 Production\\FR7 - Poitiers\\06 Production\\05. Electronique\\Documents Control lib\\Archives\\ZEN PLUS"
        n162 = Close File(refnum=w501, error in=w500) -> (path=w478:path, error out=w497:errorcluster)
        n163 = call <vilib>:"waitXms.vi"("attente (ms)"=u32 300, "errin"=w497) -> ("errout"=w490:errorcluster)  [unwired: 13 in]
        n164 = local read "Cluster"() -> (w483:T1)
        n165 = Read from Text File(file (use dialog)=w478, error in=w490) -> (text=w488:string, error out=w487:errorcluster)  [unwired: 2 in, 2 out]
        n166 = call "OP300ZP_SN_Reader.vi"("Fichier txt"=w488) -> ("SN"=w480:string)  [unwired: 10 in]
        n167 = Unbundle By Name(w483) -> ("PN"=w482:string)
        n168 = Concatenate Strings(w482, "-SN" ("chaîne"), w480) -> (w479:string)
        n169 = call "Multi_OUI_NON.vi"("errin"=w477, "errinb"=TRUE, "Tableau"=string[] ["SECU", "Next"]) -> ("errout"=w475:errorcluster, "isok?"=w474:bool)  [unwired: 7 in]
        n170 = call "OP300ZP_NouveauDossier.vi"("entrée d'erreur (pas d'erreur)"=w487, "Nom du repertoire (PN SN)"=w479, "Network before adding a new folder"=path "\\\\forseepower.com\\fr/040 Production/FR7 - Poitiers/06 Production/05. Electronique/Documents Control lib/Archives/ZEN PLUS" ("chemin de la cible (utiliser une boîte de dialogue)")) -> ("sortie d'erreur"=w486:errorcluster, "Network after adding a new folder"=w484:path)  [unwired: 7 in]
        n171 = Copy ("Copier")(8:w486, 10:w484, 11:w478) -> (0:w489:errorcluster)  [unwired: 2 in, 2 out]
        n172 = call "PvgeneratorOP300.vi"("errin"=w489, "network"=w484, "path in"=w478) -> ("sortie d'erreur"=w495:errorcluster, "network out"=w494:path, "tout bon"=w491:bool)  [unwired: 5 in, 1 out]
        n173 = call <vilib>:"POP_GOOGLE.vi"("error in"=w495, "chemin"=w494) -> ("error out"=w492:errorcluster)  [unwired: 8 in, 1 out]
        n174 = disable-structure shown="Désactivé" {
          disable-tunnel: [w510 _] -> w493
          disable-tunnel: w492 -> [w509 _]
          disable-tunnel: w491 -> [w507 _]
          frame Disabled {
            n175 = Select ("Sélectionner")(t="1", s=w507, f="0" ("cas faux")) -> (s? t:f=w504:string)
            n176 = local read "Cluster"() -> (w508:T1)
            n177 = Bundle By Name(cluster=w508, "Résultat final"=w504) -> (w503:T1)
            n178 = call "BDD_2.vi"("errin"=w509, "Cluster"=w503) -> ("error out"=w510:errorcluster)  [unwired: 8 in, 1 out]
          }
          frame Enabled {
          }
        }
        n179 = Select(t=w499, s=w474, f=w498) -> (s? t:f=w502:T4)
      }
      frame "Sealing" {
        w527 = OP300ZP_state."Montage" ("Cas OK")
        n180 = call <vilib>:"FGV_Image.vi"("Énum"=FGV."SET", "IN"="Sealing") -> ()  [unwired: 9 in, 1 out]
        n181 = call "Sealing pack"("error in (no error)"=w524) -> ("Sealing"=w518:dbl, "error out"=w533:errorcluster)  [unwired: 16 in, 1 out]
        n182 = local write "TOP"("Valeur de pression" ("TOP")) -> ()
        n183 = call <vilib>:"Application Directory.vi"() -> ("Application Directory"=w535:path)
        n184 = call <vilib>:"Read_Param.vi"("Énum"=enum16{"STR", "DBL", "U32"}."DBL", "errin"=w533, "pathin"=w535, "section"="Sealing", "key"="Max") -> ("error out"=w530:errorcluster, "dbl"=w516:dbl)  [unwired: 2 in, 3 out]
        n185 = In Range and Coerce ("Dans la gamme")(upper limit=w516, x=w518, lower limit=0.0 ("limite inférieure")) -> (In Range?=w519:bool)  [unwired: 1 out]
        n186 = call "ZenPlusOP300_refaire.vi"("image"="Refaire", "refaire"=OP300ZP_state."Sealing", "casOK"=w527, "errin"=w530, "test ok ?"=w519) -> ("errout"=w529:errorcluster, "Next"=w528:T4)  [unwired: 5 in]
        n187 = Equal?(x=w528, y=w527) -> (x = y?=w526:bool)
        n188 = case shown="Vrai" w526 {
          tunnel: w538 -> [w539 w547]
          tunnel: w537 -> [w541 w546]
          tunnel: [w541 w545] -> w536
          tunnel: w518 -> [_ w544]
          tunnel: ["0" w543] -> w513
          tunnel: [w539 w542] -> w512
          frame False {
          }
          frame True {
            n189 = Number To Decimal String(number=w544) -> (decimal integer string=w543:string)  [unwired: 1 in]
            n190 = Concatenate Strings("Sealing;" ("chaîne"), w543) -> (w549:string)
            n191 = call <vilib>:"Log_basic.vi"("errin"=w547, "date?"=TRUE, "chaîne"=w549, "in"=w546) -> ("sortie d'erreur"=w542:errorcluster, "refnum en sortie"=w545:refnum<file>)  [unwired: 6 in]
          }
        }
        n192 = local read "Cluster"() -> (w515:T1)
        n193 = Bundle By Name(cluster=w515, "Sealing"=w513) -> (w514:T1)
        n194 = local write "Cluster"(w514) -> ()
      }
      frame "Comext" {
        n195 = call <vilib>:"OUINON.vi"("errin"=w555, "image"="Comext" ("IN")) -> ("error out"=w554:errorcluster, "OUI/NON"=w551:bool)  [unwired: 8 in]
        n196 = case shown="Vrai" w551 {
          tunnel: w564 -> [w569 w581]
          tunnel: w563 -> [w568 w580]
          tunnel: [w568 w579] -> w562
          tunnel: [w569 w578] -> w561
          tunnel: [OP300ZP_state."Crash" ("OUT") w577] -> w560
          tunnel: w559 -> [_ w576]
          tunnel: [w566 w575] -> w558
          tunnel: w557 -> [_ w574]
          tunnel: w554 -> [w566 w573]
          tunnel: [w567 w572] -> w553
          tunnel: w552 -> [w567 w572]
          frame False {
          }
          frame True {
            (unwired) "Comext;" ("testname")
            w595 = OP300ZP_state."Demontage"  # Énum
            n197 = local read "PN"() -> (w592:string)
            n198 = call <vilib>:"Application Directory.vi"() -> ("Application Directory"=w594:path)
            n199 = call <vilib>:"Read_Param.vi"("Énum"=enum16{"STR", "DBL", "U32"}."U32", "errin"=w573, "pathin"=w594, "section"="DataDyn", "key"=w592) -> ("error out"=w587:errorcluster, "U32"=w590:u32)  [unwired: 2 in, 3 out]
            n200 = property on="progression" class="Gliss (strict)"(error in=w587, "Visible"=TRUE, "Value"=u8 0 ("progression")) -> (error out=w586:errorcluster)  [unwired: 1 in, 1 out]
            n201 = call <vilib>:"FGV_Image.vi"("Énum"=FGV."SET", "IN"="DataDyn") -> ()  [unwired: 9 in, 1 out]
            n202 = call "SCAN CMU.vi"("errin"=w586, "Nb modules"=w590) -> ("errout"=w605:errorcluster, "# température + #tension OK?"=w600:bool, "Vmin"=w604:dbl, "Vmax"=w603:dbl, "Tmin"=w601:dbl, "Tmax"=w602:dbl)  [unwired: 4 out]
            n203 = call "OP300ZP_Test_DataDyn.vi"("Vcell Max (V)"=w603, "MCU"=w600, "Vcell Min (V)"=w604, "appdir"=w574, "errin"=w605, "Température usine (°C)"=21.0, "Tcell Max (°C)"=w602, "Tcell Min (°C)"=w601) -> ("errout"=w599:errorcluster, "datalog"=w607:string, "pass"=w598:bool)  [unwired: 1 out]
            n204 = call <vilib>:"Log_basic.vi"("errin"=w581, "date?"=TRUE, "chaîne"=w607, "in"=w580) -> ("sortie d'erreur"=w578:errorcluster, "refnum en sortie"=w579:refnum<file>)  [unwired: 6 in]
            n205 = call "ZenPlusOP300_refaire.vi"("image"="Refaire", "refaire"=w576, "Pédale"=FALSE, "casOK"=w595, "errin"=w599, "test ok ?"=w598) -> ("errout"=w582:errorcluster, "Next"=w577:T4)  [unwired: 4 in]
            n206 = property on="progression" class="Gliss (strict)"(error in=w582, "Visible"=FALSE, "Value"=u8 0 ("progression")) -> (error out=w575:errorcluster)  [unwired: 1 in, 1 out]
          }
        }
      }
      frame "OCV" {
        w639 = OP300ZP_state."Iso" ("Cas OK")
        w629 = enum16{"STR", "DBL", "U32"}."DBL" ("Énum")
        n207 = global read "IS30%.vi" "VG IS30% ?"() -> (w608:bool)
        n208 = call "Mesure OCV"("Enable"=TRUE, "error in (no error)"=w633) -> ("Tension Bat+ Bat-"=w625:dbl, "error out"=w641:errorcluster)  [unwired: 15 in, 1 out]
        n209 = call <vilib>:"FGV_Image.vi"("Énum"=FGV."SET", "IN"="OCV") -> ()  [unwired: 9 in, 1 out]
        n210 = local write "TOP"("Meusure de la tension à vide" ("TOP")) -> ()
        n211 = Select ("Sélectionner")(t="OCV30" ("section"), s=w608, f="OCV70" ("cas faux")) -> (s? t:f=w609:string)
        n212 = call <vilib>:"Application Directory.vi"() -> ("Application Directory"=w628:path)
        n213 = call <vilib>:"Read_Param.vi"("Énum"=w629, "errin"=w641, "pathin"=w628, "section"=w609, "key"="OCVmax") -> ("error out"=w631:errorcluster, "dbl"=w627:dbl)  [unwired: 2 in, 3 out]
        n214 = call <vilib>:"Read_Param.vi"("Énum"=w629, "errin"=w631, "pathin"=w628, "section"=w609, "key"="OCVmin") -> ("error out"=w630:errorcluster, "dbl"=w626:dbl)  [unwired: 2 in, 3 out]
        n215 = In Range and Coerce(upper limit=w627, x=w625, lower limit=w626) -> (In Range?=w618:bool)  [unwired: 1 out]
        n216 = local read "Cluster"() -> (w615:T1)
        n217 = call "ZenPlusOP300_refaire.vi"("image"="Refaire", "refaire"=w612, "casOK"=w639, "errin"=w630, "test ok ?"=w618) -> ("errout"=w619:errorcluster, "Next"=w617:T4)  [unwired: 5 in]
        n218 = Equal?(x=w617, y=w639) -> (x = y?=w638:bool)
        n219 = case shown="Vrai" w638 {
          tunnel: w622 -> [w644 w650]
          tunnel: [w644 w649] -> w621
          tunnel: w624 -> [w643 w648]
          tunnel: [w643 w647] -> w620
          tunnel: w625 -> [_ w646]
          tunnel: ["0" w645] -> w613
          frame False {
          }
          frame True {
            n220 = Number To Decimal String(number=w646) -> (decimal integer string=w645:string)  [unwired: 1 in]
            n221 = Concatenate Strings("OCV;" ("chaîne"), w645) -> (w652:string)
            n222 = call <vilib>:"Log_basic.vi"("errin"=w650, "date?"=TRUE, "chaîne"=w652, "in"=w648) -> ("sortie d'erreur"=w649:errorcluster, "refnum en sortie"=w647:refnum<file>)  [unwired: 6 in]
          }
        }
        n223 = Bundle By Name(cluster=w615, "OCV"=w613) -> (w614:T1)
        n224 = local write "Cluster"(w614) -> ()
      }
    }
    n225 = Wait (ms)(milliseconds to wait=u32 200 ("attente (ms)")) -> ()  [unwired: 1 out]
    n226 = case shown="Vrai" w25 {
      selector: w25 -> [_ w32]
      frame False {
      }
      frame True {
        n227 = local write "STOP"(w32) -> ()
      }
    }
  }
  n228 = while {
    shift-right: [w662] -> _
    shift-left: errorcluster {"status"=FALSE, "code"=0, "source"=""} ("error out") -> [w659]
    stop <- w660 stop-if-true
    # "ici tu met l'image à jour si besoin"
    n229 = Wait (ms)(milliseconds to wait=u32 10 ("attente (ms)")) -> ()  [unwired: 1 out]
    n230 = call <vilib>:"FGV_Image.vi"("Énum"=FGV."GET") -> ("OUT"=w655:string)  [unwired: 10 in]
    n231 = Not Equal?(x=w655, y="") -> (x != y?=w656:bool)
    n232 = case shown="Faux" w656 {
      tunnel: [w664 w669] -> w662
      tunnel: w659 -> [w664 w668]
      tunnel: w655 -> [_ w667]
      frame False {
      }
      frame True {
        n233 = call <vilib>:"Application Directory.vi"() -> ("Application Directory"=w672:path)
        n234 = Path To String(path=w672) -> (string=w673:string)
        n235 = Concatenate Strings(w673, "\\Image\\" ("chaîne"), w667, ".jpg" ("chaîne")) -> (w671:string)
        n236 = call <vilib>:"FGV_Image.vi"("Énum"=FGV."RAZ") -> ()  [unwired: 10 in, 1 out]
        n237 = String To Path(string=w671) -> (path=w670:path)
        n238 = call <vilib>:"Read JPEG File.vi"("error in (no error)"=w668, "path to JPEG file"=w670) -> ("error out"=w669:errorcluster, "image data"=w676:T8)  [unwired: 7 in, 1 out]
        n239 = call <vilib>:"Draw Flattened Pixmap.vi"("image data"=w676) -> ("new picture"=w665:picture)  [unwired: 8 in]
        n240 = local write "DRAW"(w665) -> ()
      }
    }
    n241 = global read "VG_progressBar.vi" "progression"() -> (→"progression":u8)
    n242 = local read "STOP"() -> (w661:bool)
    n243 = Or(x=w662, y=w661) -> (x .or. y?=w660:bool)
  }
  n244 = Merge Errors(w17, w16) -> (→"errout":errorcluster)
  n245 = disable-structure shown="Activé" {
    disable-tunnel: [w677 _] -> _
    frame Disabled {
      n246 = call "Data Dynamiques"() -> ("CMU OK"=w677:bool)  [unwired: 12 in, 7 out]
    }
    frame Enabled {
    }
  }
  "STOP" <- w14
